vi "21_ВПИзмерениеТемпературы.vi"() -> ()   [LabVIEW 2016]
panel:
  out "Temperature Chart":dbl(graph)
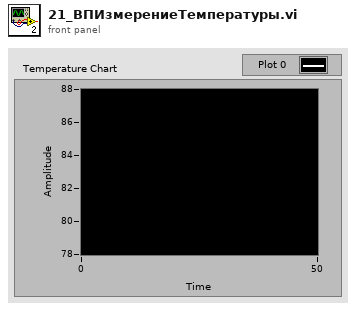
[diagram p1: front panel]
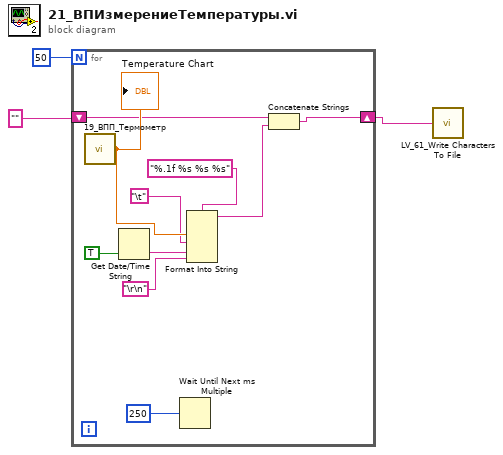
[diagram p0: block diagram]
diagram:
  n1 = for {
    N: 50 -> [_]
    shift-right: [w4] -> w1
    shift-left: "" -> [w6]
    n2 = call "19_ВПП_Термометр.vi"() -> ("Thermometer"=w10:dbl)
    "Temperature Chart" <- w10
    n3 = Get Date/Time String(want seconds? (F)=TRUE) -> (time string=w8:string)  [unwired: 2 in, 1 out]
    n4 = Wait Until Next ms Multiple(millisecond multiple=250) -> ()  [unwired: 1 out]
    n5 = Format Into String(format string="%.1f %s %s %s", w10, "\t", w8, "\r\n") -> (resulting string=w5:string)  [unwired: 2 in, 1 out]
    n6 = Concatenate Strings(w6, w5) -> (w4:string)
  }
  n7 = call "LV_61_Write Characters To File.vi"("character string"=w1) -> ()  [unwired: 4 in, 1 out]
